vi "format time stamp.vi"(8 "error in (no error)":errorcluster, 11 "Log File in":refnum<class "Log File.lvclass">) -> (0 "error out":errorcluster, 3 "Log File out":refnum<class "Log File.lvclass">)   [LabVIEW 2018, in "Log File.lvclass"]
uses:
  Log File.lvclass
  Log File.lvclass/Log File.ctl
panel:
  out "current time stamp":string
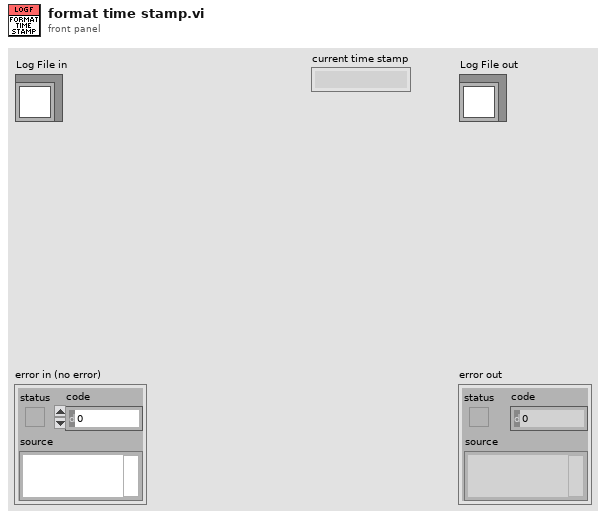
[diagram p1: front panel]
types:
  T1 = typedef "LVDateTimeRec.ctl" = cluster{"fractional second":dbl, "second":i32, "minute":i32, "hour":i32, "day of month":i32, "month":i32, "year":i32, "day of week":i32, "day of year":i32, "DST":i32}
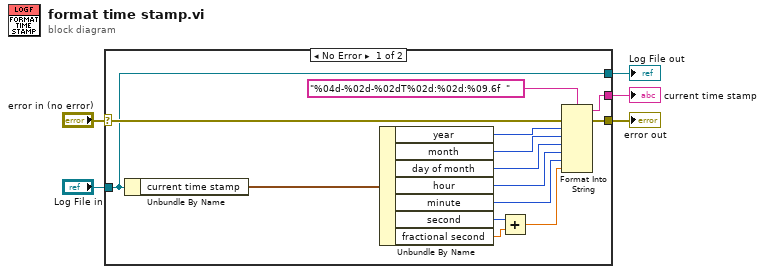
[diagram p0: block diagram]
diagram:
  n1 = case shown="No Error" "error in (no error)" {
    selector: "error in (no error)" -> [w8 w21]
    tunnel: [w10 w21] -> w4
    tunnel: [w7 w20] -> w2
    tunnel: "Log File in" -> [w7 w20]
    tunnel: [w9 _] -> w1
    frame No Error {
      n2 = Unbundle By Name(w7) -> ("current time stamp"=w6:T1)
      n3 = Unbundle By Name(w6) -> ("year"=w17:i32, "month"=w16:i32, "day of month"=w15:i32, "hour"=w14:i32, "minute"=w13:i32, "second"=w19:i32, "fractional second"=w18:dbl)
      n4 = Add(x=w19, y=w18) -> (x+y=w12:dbl)
      n5 = Format Into String(format string="%04d-%02d-%02dT%02d:%02d:%09.6f  ", error in=w8, w17, w16, w15, w14, w13, w12) -> (resulting string=w9:string, error out=w10:errorcluster)  [unwired: 1 in]
    }
    frame Error {
    }
  }
  "error out" <- w4
  "Log File out" <- w2
  "current time stamp" <- w1
